vi "GetSL2AD_VI_dllPath.vi"(11 "dll_path":path) -> (0 "error":errorcluster, 2 "found?":bool, 3 "Path":path)   [LabVIEW 2020]
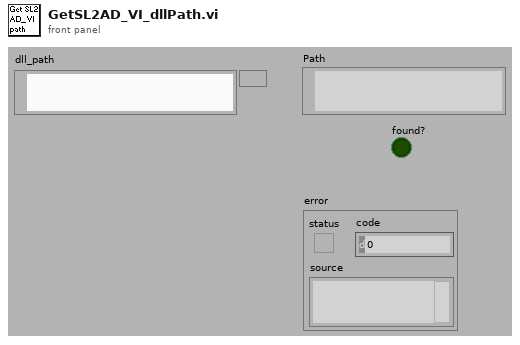
[diagram p1: front panel]
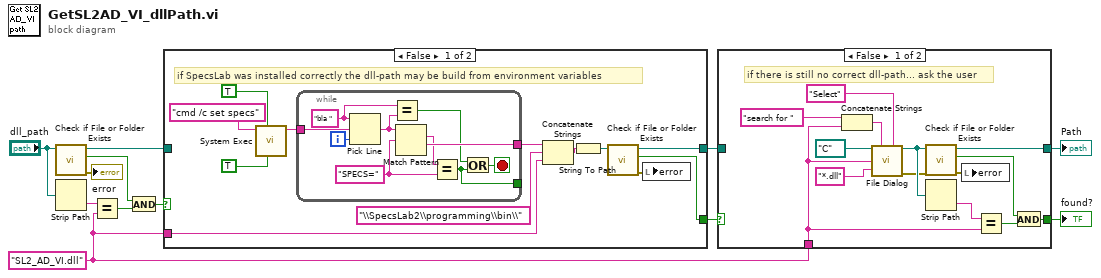
[diagram p0: block diagram]
diagram:
  w1 = "SL2_AD_VI.dll" ("default name")
  n1 = call <vilib>:"Check if File or Folder Exists.vi"("path"="dll_path") -> ("error out"=→"error":errorcluster, "file or folder exists?"=w9:bool, "dup path"=w6:path)  [unwired: 8 in]
  n2 = Strip Path(path="dll_path") -> (name=w11:string)  [unwired: 1 out]
  n3 = Equal?(x=w11, y=w1) -> (x = y?=w10:bool)
  n4 = And(x=w9, y=w10) -> (x .and. y?=w7:bool)
  n5 = case shown="False" w7 {
    selector: w7 -> [_ w35]
    tunnel: [w17 w36] -> w4
    tunnel: w6 -> [_ w36]
    tunnel: [w16 w35] -> w5
    tunnel: w1 -> [w13 _]
    frame False {
      # "if SpecsLab was installed correctly the dll-path may be build from environment variables"
      n6 = call <vilib>:"System Exec.vi"("run minimized? (F)"=TRUE, "wait until completion? (T)"=TRUE, "command line"="cmd /c set specs") -> ("standard output"=w21:string)  [unwired: 5 in, 3 out]
      n7 = while {
        tunnel: w21 -> [w34]
        tunnel: [w30] -> w22
        tunnel: [w25] -> _
        i -> [w33]
        stop <- w27 stop-if-true
        w32 = "bla " ("regular expression")
        w28 = "SPECS=" ("regular expression")
        n8 = Pick Line(string ("")=w32, multi-line string=w34, line index=w33) -> (output string=w31:string)
        n9 = Equal?(x=w32, y=w31) -> (x = y?=w26:bool)
        n10 = Match Pattern(string=w31, regular expression=w28) -> (match substring=w29:string, after substring=w30:string)  [unwired: 1 in, 2 out]
        n11 = Equal?(x=w29, y=w28) -> (x = y?=w25:bool)
        n12 = Or(x=w26, y=w25) -> (x .or. y?=w27:bool)
      }
      n13 = Concatenate Strings(w22, "\\SpecsLab2\\programming\\bin\\", w13) -> (w24:string)
      n14 = String To Path(string=w24) -> (path=w14:path)
      n15 = call <vilib>:"Check if File or Folder Exists.vi"("path"=w14) -> ("error out"=w15:errorcluster, "file or folder exists?"=w16:bool, "dup path"=w17:path)  [unwired: 8 in]
      n16 = local write "error"(w15) -> ()
    }
    frame True {
      # "a correct dll-path was passed"
    }
  }
  n17 = case shown="False" w5 {
    selector: w5 -> [_ w51]
    tunnel: [w45 w52] -> w3
    tunnel: w4 -> [_ w52]
    tunnel: [w44 w51] -> w2
    tunnel: w1 -> [w37 _]
    frame False {
      # "if there is still no correct dll-path... ask the user"
      n18 = Concatenate Strings("search for " ("prompt"), w37) -> (w38:string)
      n19 = call "File Dialog"("start path"=path "C:/", "prompt"=w38, "button label"="Select", "default name"=w37, "pattern (all files)"="*.dll") -> ("selected path"=w42:path, "error out"=w40:errorcluster)  [unwired: 7 in, 2 out]
      n20 = call <vilib>:"Check if File or Folder Exists.vi"("error in (no error)"=w40, "path"=w42) -> ("error out"=w41:errorcluster, "file or folder exists?"=w43:bool, "dup path"=w45:path)  [unwired: 7 in]
      n21 = Strip Path(path=w42) -> (name=w47:string)  [unwired: 1 out]
      n22 = local write "error"(w41) -> ()
      n23 = Equal?(x=w47, y=w37) -> (x = y?=w46:bool)
      n24 = And(x=w43, y=w46) -> (x .and. y?=w44:bool)
    }
    frame True {
      # "a correct dll-path was passed"
    }
  }
  "Path" <- w3
  "found?" <- w2
